vi "velocity-subvi-v2.vi"(3 "Axis Select":u8(slide)=1 min=1 max=4 step=1 scale=1.0..4.0, 4 "Velocity unit":T1(ring)=enum."mm/sec", 5 "Velocity":dbl=6000.0) -> (0 "Boolean":bool, 1 "Velocity unit":string, 2 "Velocity Corrected":dbl=6000.0)   [LabVIEW 2009]
uses:
  Instance           1 22Saved   velocity-subvi .vi
  Instance           3 22Saved   velocity-subvi .vi
  Instance           2 22Saved   velocity-subvi .vi
  Instance           4 22Saved   velocity-subvi .vi
  Instance           5 22Saved   velocity-subvi .vi
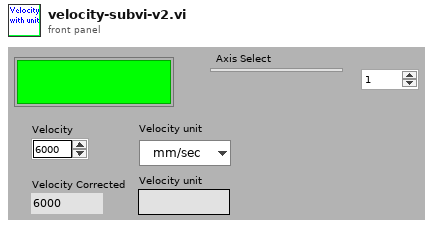
[diagram p1: front panel]
types:
  T1 = enum16{"fs/sec", "ps/sec", "um/sec", "mm/sec", "counts/sec"}
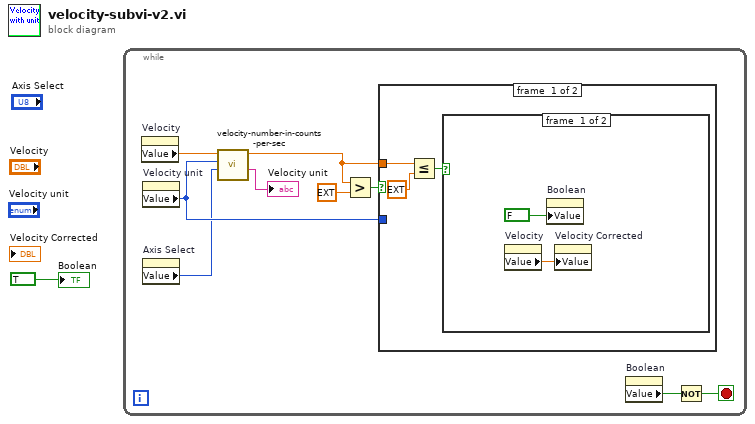
[diagram p0: block diagram]
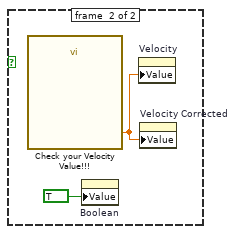
[diagram p2: hidden frame]
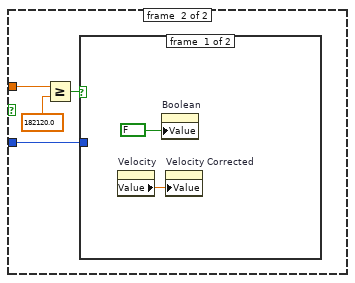
[diagram p3: hidden frame]
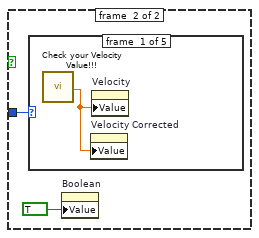
[diagram p4: hidden frame]
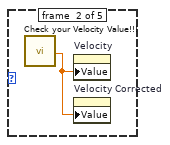
[diagram p5: hidden frame]
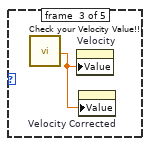
[diagram p6: hidden frame]
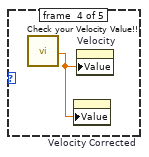
[diagram p7: hidden frame]
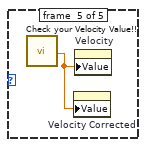
[diagram p8: hidden frame]
diagram:
  n1 = while {
    stop <- w8 stop-if-true
    n2 = property on="Velocity" class="DigNum (strict)"() -> ("Value"=w5:dbl)  [unwired: 2 in, 2 out]
    n3 = property on="Velocity unit" class="Enum (strict)"() -> ("Value"=w3:T1)  [unwired: 2 in, 2 out]
    n4 = property on="Axis Select" class="Slide (strict)"() -> ("Value"=w2:u8)  [unwired: 2 in, 2 out]
    n5 = call "velocity-number-in-counts-per-sec.vi"("Axis Select"=w2, "unit"=w3, "velocity"=w5) -> ("unit"=→"Velocity unit":string, "counts"=w7:dbl)  [unwired: 7 in]
    n6 = Greater?(x=w7, y=ext 0.0) -> (0:w9:bool)
    n7 = case shown="True" w9 {
      tunnel: w7 -> [w11 w19]
      tunnel: w3 -> [_ w18]
      frame #0 {
        n8 = Less Or Equal?(x=w11, y=ext 0.0) -> (x <= y?=w12:bool)
        n9 = case shown="True" w12 {
          frame #0 {
            n10 = property on="Velocity" class="DigNum (strict)"() -> ("Value"=w15:dbl)  [unwired: 2 in, 2 out]
            n11 = property on="Boolean" class="Bool (strict)"("Value"=FALSE) -> ()  [unwired: 2 in, 2 out]
            n12 = property on="Velocity Corrected" class="DigNum (strict)"("Value"=w15) -> ()  [unwired: 2 in, 2 out]
          }
          frame #1 {
            n13 = call "Check your Velocity Value!!!"() -> ("Velocity"=w16:dbl)  [unwired: 17 in, 2 out]
            n14 = property on="Boolean" class="Bool (strict)"("Value"=TRUE) -> ()  [unwired: 2 in, 2 out]
            n15 = property on="Velocity" class="DigNum (strict)"("Value"=w16) -> ()  [unwired: 2 in, 2 out]
            n16 = property on="Velocity Corrected" class="DigNum (strict)"("Value"=w16) -> ()  [unwired: 2 in, 2 out]
          }
        }
      }
      frame #1 {
        n17 = Greater Or Equal?(x=w19, y=182120.0) -> (x >= y?=w20:bool)
        n18 = case shown="True" w20 {
          tunnel: w18 -> [_ w25]
          frame #0 {
            n19 = property on="Velocity" class="DigNum (strict)"() -> ("Value"=w23:dbl)  [unwired: 2 in, 2 out]
            n20 = property on="Boolean" class="Bool (strict)"("Value"=FALSE) -> ()  [unwired: 2 in, 2 out]
            n21 = property on="Velocity Corrected" class="DigNum (strict)"("Value"=w23) -> ()  [unwired: 2 in, 2 out]
          }
          frame #1 {
            n22 = case shown="\"counts/sec\", Default" w25 {
              frame #0 {
                n23 = call "Check your Velocity Value!!!"() -> ("Velocity"=w26:dbl)  [unwired: 17 in, 2 out]
                n24 = property on="Velocity Corrected" class="DigNum (strict)"("Value"=w26) -> ()  [unwired: 2 in, 2 out]
                n25 = property on="Velocity" class="DigNum (strict)"("Value"=w26) -> ()  [unwired: 2 in, 2 out]
              }
              frame #1 {
                n26 = call "Check your Velocity Value!!!"() -> ("Velocity"=w27:dbl)  [unwired: 17 in, 2 out]
                n27 = property on="Velocity" class="DigNum (strict)"("Value"=w27) -> ()  [unwired: 2 in, 2 out]
                n28 = property on="Velocity Corrected" class="DigNum (strict)"("Value"=w27) -> ()  [unwired: 2 in, 2 out]
              }
              frame #2 {
                n29 = call "Check your Velocity Value!!!"() -> ("Velocity"=w28:dbl)  [unwired: 17 in, 2 out]
                n30 = property on="Velocity" class="DigNum (strict)"("Value"=w28) -> ()  [unwired: 2 in, 2 out]
                n31 = property on="Velocity Corrected" class="DigNum (strict)"("Value"=w28) -> ()  [unwired: 2 in, 2 out]
              }
              frame #3 {
                n32 = call "Check your Velocity Value!!!"() -> ("Velocity"=w29:dbl)  [unwired: 17 in, 2 out]
                n33 = property on="Velocity Corrected" class="DigNum (strict)"("Value"=w29) -> ()  [unwired: 2 in, 2 out]
                n34 = property on="Velocity" class="DigNum (strict)"("Value"=w29) -> ()  [unwired: 2 in, 2 out]
              }
              frame #4 {
                n35 = call "Check your Velocity Value!!!"() -> ("Velocity"=w30:dbl)  [unwired: 17 in, 2 out]
                n36 = property on="Velocity Corrected" class="DigNum (strict)"("Value"=w30) -> ()  [unwired: 2 in, 2 out]
                n37 = property on="Velocity" class="DigNum (strict)"("Value"=w30) -> ()  [unwired: 2 in, 2 out]
              }
            }
            n38 = property on="Boolean" class="Bool (strict)"("Value"=TRUE) -> ()  [unwired: 2 in, 2 out]
          }
        }
      }
    }
    n39 = property on="Boolean" class="Bool (strict)"() -> ("Value"=w4:bool)  [unwired: 2 in, 2 out]
    n40 = Not(x=w4) -> (.not. x?=w8:bool)
  }
  "Boolean" <- TRUE
